vi "Build.vi"(9 "XYZTheta":dbl[](array[numeric]), 10 "text file":dbl[][](array[numeric]), 11 "Sensor Dispense in":refnum<class "Sensor Dispense.lvclass">) -> (3 "Sensor Dispense out":refnum<class "Sensor Dispense.lvclass">)   [LabVIEW 2020, in "Sensor Dispense.lvclass"]
uses:
  Projects/Sensor Dispense.lvclass
  C:/Users/HEP/Documents/GitHub/UCSB-Gantry-HEP/Classes/Routine/Dispense/Dispense.lvclass
  Projects/Sensor Dispense.lvclass/Sensor Dispense.ctl
  <vilib>/Analysis/coordinate.llb/2D Cartesian Coordinate Rotation (Scalar).vi
  <vilib>/Analysis/NI_AALPro.lvlib
panel:
  out "CW/CCW":dbl[](array[numeric])
  out "CW/CCW":dbl[](array[numeric])
  out "endpoints 2":dbl[][](array[numeric])
  out "endpoints":dbl[][](array[numeric])
  out "data":T1(array[cluster])
  out "cell count":dbl[](array[numeric])
  out "centers":dbl[][](array[numeric])
  # "[x1,y1,x2,y2]"
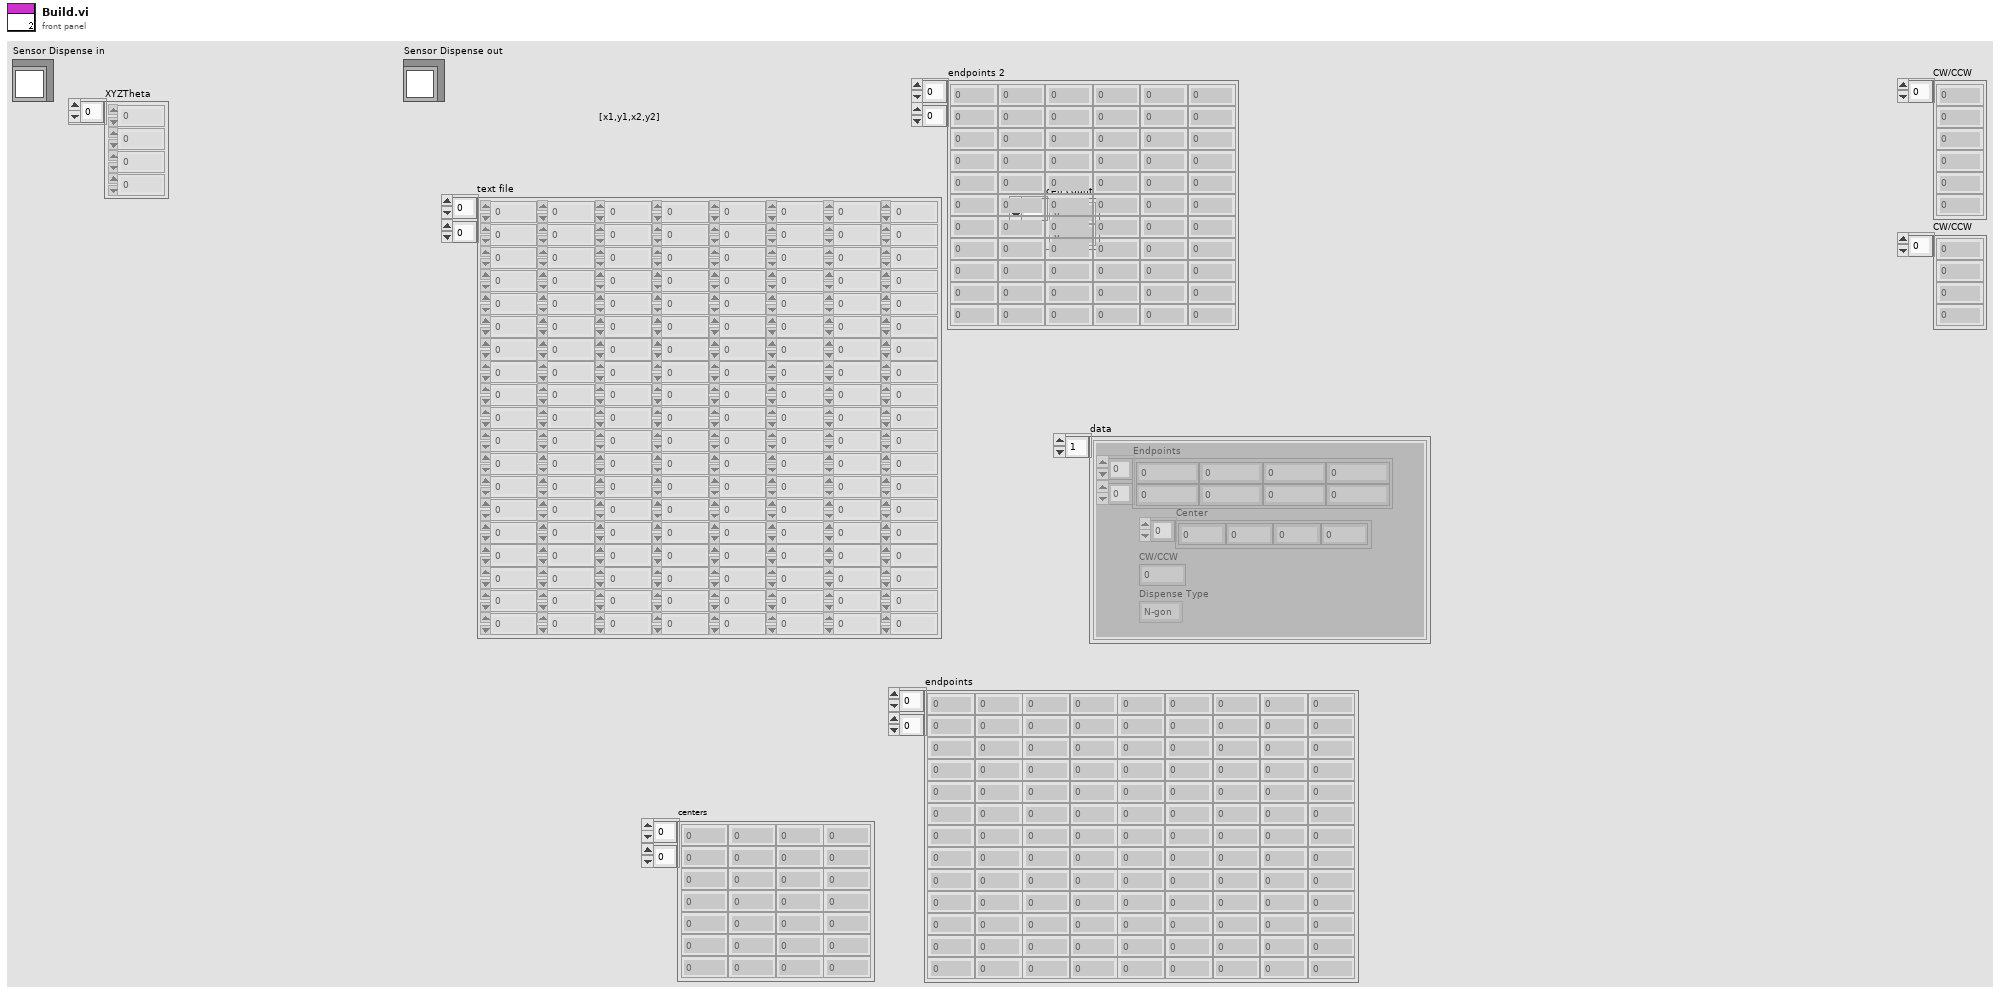
[diagram p1: front panel]
types:
  T1 = cluster{"Endpoints":dbl[][], "Center":dbl[], "CW/CCW":dbl, "Dispense Type":enum16{"N-gon", "Square", "Arc", "Dot", "Line", "Circle"}}[]
  T2 = enum16{"N-gon", "Square", "Arc", "Dot", "Line", "Circle"}
  T3 = cluster{"Endpoints":dbl[][], "Center":dbl[], "CW/CCW":dbl, "Dispense Type":enum16{"N-gon", "Square", "Arc", "Dot", "Line", "Circle"}}
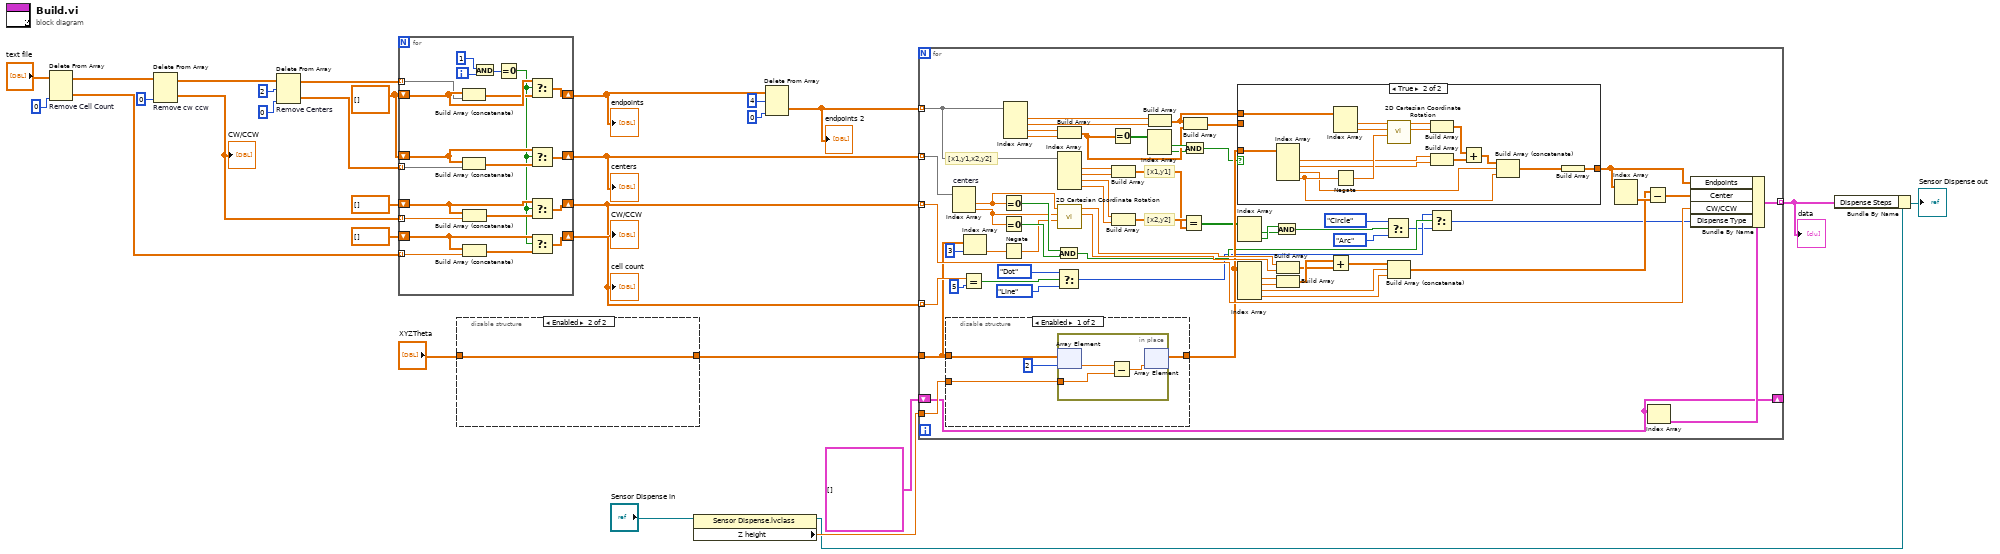
[diagram p0: block diagram]
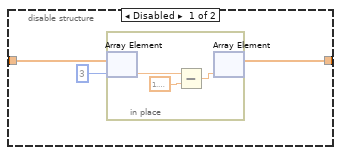
[diagram p2: hidden frame]
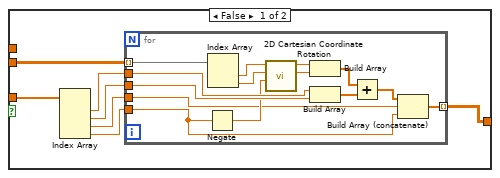
[diagram p4: hidden frame]
diagram:
  w26 = dbl[][] []
  n1 = Delete From Array "Remove Cell Count"(array="text file", index (col)=0) -> (deleted portion=w20:dbl[], array with subset deleted=w22:dbl[][])  [unwired: 2 in]
  n2 = Delete From Array "Remove cw ccw"(array=w22, index (col)=0 ("disabled index (col)")) -> (deleted portion=w2:dbl[], array with subset deleted=w19:dbl[][])  [unwired: 2 in]
  "CW/CCW" <- w2
  n3 = Delete From Array "Remove Centers"(array=w19, length=2, index (col)=0) -> (deleted portion=w15:dbl[][], array with subset deleted=w16:dbl[][])  [unwired: 1 in]
  n4 = for {
    tunnel: w16 -> [w45] mode=indexing
    shift-right: [w43] -> w9
    shift-left: w26 -> [w46]
    tunnel: w15 -> [w42] mode=indexing
    shift-right: [w39] -> w27
    shift-left: w26 -> [w40]
    tunnel: w20 -> [w38] mode=indexing
    shift-right: [w35] -> w24
    shift-left: dbl[] [] -> [w37]
    shift-right: [w30] -> w1
    shift-left: dbl[] [] -> [w33]
    tunnel: w2 -> [w34] mode=indexing
    i -> [w48]
    n5 = Build Array (concatenate)(w46, w45) -> (w44:dbl[][])
    n6 = Build Array (concatenate)(w40, w42) -> (w41:dbl[][])
    n7 = Build Array (concatenate)(w33, w34) -> (w32:dbl[])
    n8 = Build Array (concatenate)(w37, w38) -> (w36:dbl[])
    n9 = And(x=1, y=w48) -> (x .and. y?=w47:i32)
    n10 = Equal To 0?(x=w47) -> (x = 0?=w31:bool)
    n11 = Select(t=w46, s=w31, f=w44) -> (s? t:f=w43:dbl[][])
    n12 = Select(t=w40, s=w31, f=w41) -> (s? t:f=w39:dbl[][])
    n13 = Select(t=w33, s=w31, f=w32) -> (s? t:f=w30:dbl[])
    n14 = Select(t=w37, s=w31, f=w36) -> (s? t:f=w35:dbl[])
  }
  "centers" <- w27
  "cell count" <- w24
  "endpoints" <- w9
  "CW/CCW" <- w1
  n15 = disable-structure shown="Enabled" {
    disable-tunnel: "XYZTheta" -> [w52 w56]
    disable-tunnel: [w50 w56] -> w4
    frame Disabled {
      n16 = in-place {
        n17 = in-place-array #1(w52, 3) -> (w55:dbl)
        n18 = Subtract(x=w55, y=1.5707963267948966) -> (x-y=w53:dbl)
        n19 = in-place-array #1(w53) -> (w50:dbl[])  [unwired: 1 out]
      }
    }
    frame Enabled {
    }
  }
  n20 = property class="Sensor Dispense.lvclass"(reference="Sensor Dispense in") -> (reference out=w12:refnum<class "Sensor Dispense.lvclass">, "Z height"=w29:dbl)  [unwired: 1 in, 1 out]
  n21 = Delete From Array(array=w9, length=4, index (col)=0 ("disabled index (col)")) -> (deleted portion=w6:dbl[][])  [unwired: 1 in, 1 out]
  "endpoints 2" <- w6
  n22 = for {
    tunnel: w6 -> [w69] mode=indexing
    tunnel: w4 -> [w82]
    tunnel: w29 -> [w117]
    tunnel: w27 -> [w116] mode=indexing
    tunnel: w1 -> [w115] mode=indexing
    tunnel: w24 -> [w114] mode=indexing
    shift-right: [w93] -> _
    shift-left: T1 [] ("Dispense Steps") -> [w93]
    tunnel: [w113] -> w11 mode=indexing
    # "[x2,y2]"
    # "[x1,y1]"
    # "[x1,y1,x2,y2]"
    n23 = disable-structure shown="Enabled" {
      disable-tunnel: w117 -> [w121 _]
      disable-tunnel: [w119 w125] -> w110
      disable-tunnel: w82 -> [w118 w125]
      frame Enabled {
        n24 = in-place {
          in-place-border: w121 -> [w123]
          n25 = in-place-array #2(w118, 2) -> (w124:dbl)
          n26 = Subtract(x=w124, y=w123) -> (x-y=w122:dbl)
          n27 = in-place-array #2(w122) -> (w119:dbl[])  [unwired: 1 out]
        }
      }
      frame Disabled {
      }
    }
    n28 = Index Array "centers"(array=w116) -> (element #1=w100:dbl, element #2=w99:dbl)  [unwired: 2 in]
    n29 = Equal?(x=w114, y=5) -> (x = y?=w95:bool)
    n30 = Index Array(array=w82, index=3) -> (element=w81:dbl)
    n31 = Equal To 0?(x=w100) -> (x = 0?=w101:bool)
    n32 = Equal To 0?(x=w99) -> (x = 0?=w102:bool)
    n33 = Negate(x=w81) -> (-x=w80:dbl)
    n34 = Index Array(array=w69) -> (element #1=w67:dbl, element #2=w66:dbl, element #3=w65:dbl, element #4=w64:dbl)  [unwired: 4 in]
    n35 = And(x=w101, y=w102) -> (x .and. y?=w78:bool)
    n36 = Select(t=T2."Dot" ("Dispense Type"), s=w95, f=T2."Line" ("Dispense Type")) -> (s? t:f=w77:T2)
    n37 = Build Array(w65, w64) -> (w61:dbl[])
    n38 = Index Array(array=w69) -> (element #1=w75:dbl, element #2=w74:dbl, element #3=w92:dbl, element #4=w91:dbl)  [unwired: 4 in]
    n39 = call-poly <vilib>:"2D Cartesian Coordinate Rotation.vi"("theta"=w80, "y"=w99, "x"=w100) -> ("y out"=w111:dbl, "x out"=w112:dbl)  [unwired: 6 in, 1 out]
    n40 = Equal To 0?(x=w61) -> (x = 0?=w60:bool[])
    n41 = Build Array(w75, w74) -> (w89:dbl[])
    n42 = Build Array(w92, w91) -> (w90:dbl[])
    n43 = Index Array(array=w60) -> (element #1=w62:bool, element #2=w58:bool)  [unwired: 2 in]
    n44 = Build Array(w67, w66) -> (w57:dbl[])
    n45 = Equal?(x=w90, y=w89) -> (x = y?=w86:bool[])
    n46 = And(x=w62, y=w58) -> (x .and. y?=w59:bool)
    n47 = Build Array(w57, w61) -> (w63:dbl[][])
    n48 = case shown="True" w59 {
      tunnel: w110 -> [w132 w159]
      tunnel: [w131 w147] -> w73
      tunnel: w63 -> [w130 _]
      tunnel: w57 -> [_ w162]
      frame False {
        n49 = Index Array(array=w132) -> (element #1=w129:dbl, element #2=w128:dbl, element #3=w126:dbl, element #4=w127:dbl)  [unwired: 4 in]
        n50 = for {
          tunnel: w130 -> [w146] mode=indexing
          tunnel: w129 -> [w143]
          tunnel: w128 -> [w142]
          tunnel: [w133] -> w131 mode=indexing
          tunnel: w127 -> [w134]
          tunnel: w126 -> [w135]
          n51 = Negate(x=w134) -> (-x=w137:dbl)
          n52 = Index Array(array=w146) -> (element #1=w145:dbl, element #2=w144:dbl)  [unwired: 2 in]
          n53 = call-poly <vilib>:"2D Cartesian Coordinate Rotation.vi"("theta"=w137, "y"=w144, "x"=w145) -> ("y out"=w140:dbl, "x out"=w141:dbl)  [unwired: 6 in, 1 out]
          n54 = Build Array(w141, w140) -> (w139:dbl[])
          n55 = Build Array(w143, w142) -> (w138:dbl[])
          n56 = Add(x=w139, y=w138) -> (x+y=w136:dbl[])
          n57 = Build Array (concatenate)(w136, w135, w134) -> (w133:dbl[])
        }
      }
      frame True {
        n58 = Index Array(array=w159) -> (element #1=w155:dbl, element #2=w154:dbl, element #3=w150:dbl, element #4=w151:dbl)  [unwired: 4 in]
        n59 = Index Array(array=w162) -> (element #1=w161:dbl, element #2=w160:dbl)  [unwired: 2 in]
        n60 = Negate(x=w151) -> (-x=w158:dbl)
        n61 = call-poly <vilib>:"2D Cartesian Coordinate Rotation.vi"("theta"=w158, "y"=w160, "x"=w161) -> ("y out"=w156:dbl, "x out"=w157:dbl)  [unwired: 6 in, 1 out]
        n62 = Build Array(w157, w156) -> (w152:dbl[])
        n63 = Build Array(w155, w154) -> (w153:dbl[])
        n64 = Add(x=w152, y=w153) -> (x+y=w149:dbl[])
        n65 = Build Array (concatenate)(w149, w150, w151) -> (w148:dbl[])
        n66 = Build Array(w148) -> (w147:dbl[][])
      }
    }
    n67 = Index Array(array=w86) -> (element #1=w84:bool, element #2=w85:bool)  [unwired: 2 in]
    n68 = Index Array(array=w110) -> (element #1=w109:dbl, element #2=w106:dbl, element #3=w104:dbl, element #4=w103:dbl)  [unwired: 4 in]
    n69 = And(x=w85, y=w84) -> (x .and. y?=w83:bool)
    n70 = Build Array(w112, w111) -> (w107:dbl[])
    n71 = Build Array(w109, w106) -> (w108:dbl[])
    n72 = Add(x=w108, y=w107) -> (x+y=w105:dbl[])
    n73 = Select(t=T2."Circle" ("Dispense Type"), s=w83, f=T2."Arc" ("Dispense Type")) -> (s? t:f=w76:T2)
    n74 = Build Array (concatenate)(w105, w104, w103) -> (w71:dbl[])
    n75 = Select(t=w77, s=w78, f=w76) -> (s? t:f=w68:T2)
    n76 = Index Array(array=w73) -> (element=w72:dbl[])  [unwired: 2 in]
    n77 = Subtract(x=w71, y=w72) -> (x-y=w70:dbl[])
    n78 = Index Array(array=w93) -> (element=w94:T3)  [unwired: 1 in]
    n79 = Bundle By Name(cluster=w94, "Endpoints"=w73, "Center"=w70, "CW/CCW"=w115, "Dispense Type"=w68) -> (w113:T3)
  }
  "data" <- w11
  n80 = Bundle By Name(cluster=w12, "Dispense Steps"=w11) -> (→"Sensor Dispense out":refnum<class "Sensor Dispense.lvclass">)
